vi "supportedFunctions.vi"(0 "String":string) -> (1 "regular expression":string, 2 "Priority":i32)   [LabVIEW 2014]
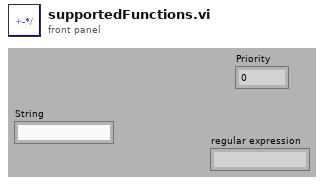
[diagram p1: front panel]
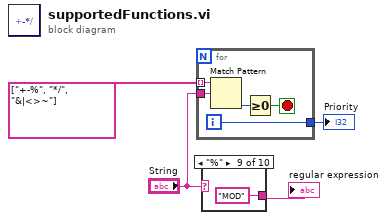
[diagram p0: block diagram]
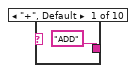
[diagram p2: hidden frame]
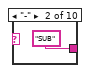
[diagram p3: hidden frame]
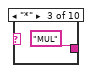
[diagram p4: hidden frame]
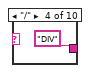
[diagram p5: hidden frame]
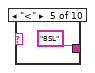
[diagram p6: hidden frame]
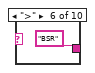
[diagram p7: hidden frame]
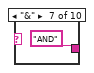
[diagram p8: hidden frame]
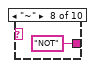
[diagram p9: hidden frame]
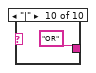
[diagram p10: hidden frame]
diagram:
  n1 = for {
    tunnel: "String" -> [w9]
    tunnel: string[] ["+-%", "*/", "&|<>~"] -> [w8] mode=indexing
    tunnel: [w5] -> w1
    i -> [w5]
    stop <- w6 stop-if-true
    n2 = Match Pattern(string=w8, regular expression=w9) -> (offset past match=w7:i32)  [unwired: 1 in, 3 out]
    n3 = Greater Or Equal To 0?(x=w7) -> (x >= 0?=w6:bool)
  }
  "Priority" <- w1
  n4 = case shown="\"%\"" "String" {
    tunnel: ["ADD" ("regular expression") "SUB" ("regular expression") "MUL" ("regular expression") "DIV" ("regular expression") "BSL" ("regular expression") "BSR" ("regular expression") "AND" ("regular expression") "NOT" ("regular expression") "MOD" ("regular expression") "OR" ("regular expression")] -> w4
    frame "+", Default {
    }
    frame "-" {
    }
    frame "*" {
    }
    frame "/" {
    }
    frame "<" {
    }
    frame ">" {
    }
    frame "&" {
    }
    frame "~" {
    }
    frame "%" {
    }
    frame "|" {
    }
  }
  "regular expression" <- w4
